vi "Script Empty System Definition.vi"(8 "error in":errorcluster, 11 "System Definition Name":string) -> (0 "error out":errorcluster, 3 "System Definition Path":path)   [LabVIEW 2020]
doc: "setUp runs prior to the test method during test execution. Use this method to initialize any object data required by your tests."
uses:
  NationalInstruments.VeriStand.SystemDefinitionAPI
  niveristand-custom-device-testing-tools/VeriStandTestUtilities/VeriStandTestUtilities.lvlib
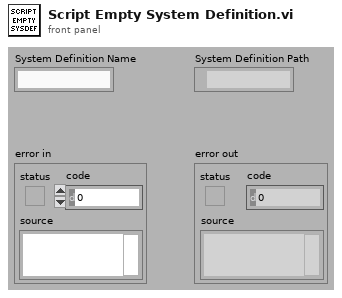
[diagram p1: front panel]
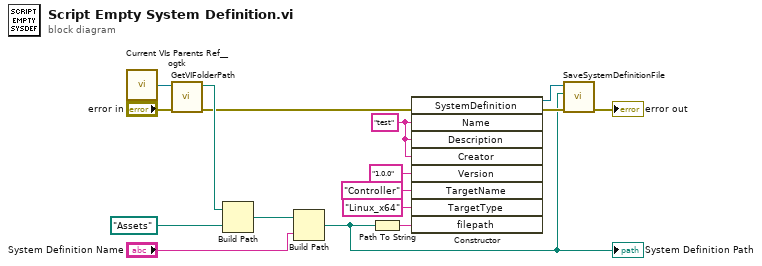
[diagram p0: block diagram]
diagram:
  w11 = "test" ("Name")
  n1 = call <userlib>:"Current VIs Parents Ref__ogtk.vi"() -> ("Calling VI's Reference"=w16:refnum<vi>)  [unwired: 2 in]
  n2 = call "GetVIFolderPath.vi"("error in (no error)"="error in", "VI Reference in"=w16) -> ("error out"=w7:errorcluster, "VI Folder Path out"=w14:path)  [unwired: 8 in]
  n3 = Build Path(base path=w14, name or relative path=path "Assets" ("Absolute or Relative Path")) -> (appended path=w6:path)
  n4 = Build Path(base path=w6, name or relative path="System Definition Name") -> (appended path=w3:path)
  "System Definition Path" <- w3
  n5 = Path To String(path=w3) -> (string=w12:string)
  n6 = constructor class="SystemDefinition"(error in=w7, "Name"=w11, "Description"=w11, "Creator"=w11, "Version"="1.0.0", "TargetName"="Controller", "TargetType"="Linux_x64", "filepath"=w12) -> (reference out=w4:refnum<k24>, error out=w5:errorcluster)  [unwired: 2 in, 8 out]
  n7 = call "SaveSystemDefinitionFile.vi"("error in (no error)"=w5, "System Definition File in"=w3, "System Definition Reference in"=w4) -> ("error out"=→"error out":errorcluster)  [unwired: 7 in, 1 out]
